vi "Configure Active DUT SIM Slot Profile.vi"(8 "error in (no error)":errorcluster, 9 "SIM Profile (\"SIMProfile\")":string="SIMProfile", 10 "SIM Slot (1)":i32=1, 11 "VISA resource name":refnum<visa-resource-name>) -> (0 "error out":errorcluster, 3 "VISA resource name out":refnum<visa-resource-name>)   [LabVIEW 2015, in "Rohde&Schwarz CMXP Base.lvlib"]
doc: "Assigns a SIM profile to a SIM slot of the active DUT.\n\nAttribute:\nRSCMXPBASE_ATTR_ACTIVE_DUT_SIM_SLOT_PROFILE\n\nRemote-control command:\n[CONFigure:]DUT:MODem<ModemIdx>:SIMSlot:SIMProfile"
uses:
  <instrlib>/Rohde&Schwarz CMXP Base/Rohde&Schwarz CMXP Base.lvlib
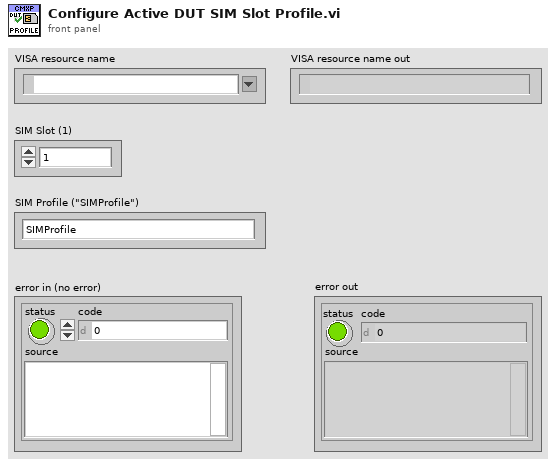
[diagram p1: front panel]
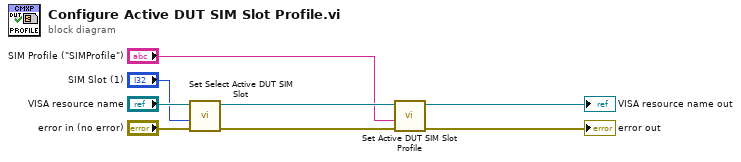
[diagram p0: block diagram]
diagram:
  n1 = call "Set Select Active DUT SIM Slot"("error in (no error)"="error in (no error)", "Select Active DUT SIM Slot (0)"="SIM Slot (1)", "instrument handle"="VISA resource name") -> ("error out"=w3:errorcluster, "instrument handle out"=w4:refnum<visa-resource-name>)  [unwired: 7 in]
  n2 = call "Set Active DUT SIM Slot Profile"("error in (no error)"=w3, "Active DUT SIM Slot Profile ()"="SIM Profile (\"SIMProfile\")", "instrument handle"=w4) -> ("error out"=→"error out":errorcluster, "instrument handle out"=→"VISA resource name out":refnum<visa-resource-name>)  [unwired: 7 in]
